vi "Fpga-Counter-U16.vi"(10 "d_mcs_i\\IO_BUS_read_strobe":bool) -> (2 "Numeric":u16)   [LabVIEW 2017]
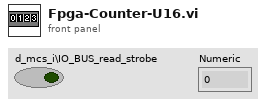
[diagram p1: front panel]
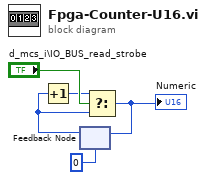
[diagram p0: block diagram]
diagram:
  n1 = feedback #1(u16 0) -> (w3:u16)
  n2 = Increment(x=w3) -> (x+1=w4:u16)
  n3 = Select(t=w4, s="d_mcs_i\\IO_BUS_read_strobe", f=w3) -> (s? t:f=w1:u16)
  "Numeric" <- w1
  n4 = feedback-in #1(w1) -> ()
